vi "LINX - Servo 1 Channel my.vi"() -> ()   [LabVIEW 2017]
doc: "This example demonstrates how to control a servo using LINX."
uses:
  <vilib>/MakerHub/LINX/Public/Utilities/Open Serial.vi
  <vilib>/MakerHub/LINX/Public/Sensors/Motion/Servo/Servo Open One Channel.vi
  <vilib>/MakerHub/LINX/Public/Sensors/Motion/Servo/Servo Set Pulse Width One Channel.vi
  <vilib>/MakerHub/LINX/Public/Sensors/Motion/Servo/Servo Close One Channel.vi
  <vilib>/express/express arith-compare/Formula/XNode/ExpressFormulaBlockNode.xnode
  <vilib>/MakerHub/LINX/LMH-LINX.lvlib
  <vilib>/MakerHub/LINX/Public/Sensors/Motion/Servo/Servo.lvlib
panel:
  out "Boolean 5":bool
  out "Boolean 4":bool
  out "Boolean 3":bool
  out "Boolean 2":bool
  out "Boolean":bool
  in  "Numeric Control 4":dbl
  in  "Numeric Control 3":dbl
  in  "Soak method":string(combo)
  out "Thermometer 2":dbl(slide) scale=0.0..100.0
  out "Thermometer":dbl(slide) scale=0.0..100.0
  out "mov_ult":dbl
  out "mov1":dbl
  out "mov_for":dbl
  in  "Setpoint":dbl
  in  "Setpoint":dbl
  out "Numeric Control 2":i32
  in  "Numeric Control":i32
  out "Position":dbl(knob) scale=500.0..2500.0
  in  "Right delay":dbl
  in  "Left delay":dbl
  in  "Maximum angle":dbl(knob) scale=500.0..2500.0
  in  "Minimum angle":dbl(knob) scale=500.0..2500.0
  in  "Right velocity":dbl
  in  "Left velocity":dbl
  in  "Servo Channel":u8=2
  in  "Stop Button":bool
  in  "Serial Port":refnum<visa-resource-name>
  # "Servo Position \n(Pulse Width uS)"
  # "Servo Velocity \n(Pulse Width uS)"
  # "Hot Box"
  # "LINX Device Settings"
  # "Current temperature 1"
  # "Cycles"
  # "Servo Delay"
  # "Cold Box"
  # "Current temperature 2"
  # "Servo Live"
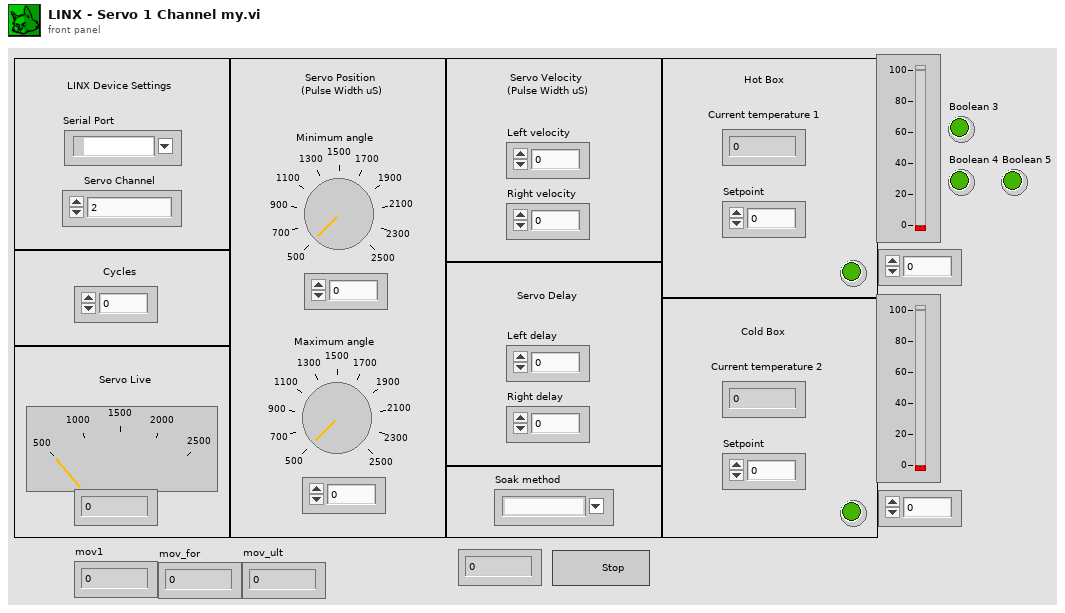
[diagram p1: front panel]
types:
  T1 = typedef "LMH-LINX.lvlib/LINX Ref.ctl" = cluster{"IO":T2, "Interface":T3, "LINX Device Config":T4}
  T2 = typedef "LMH-LINX.lvlib/Platform.ctl" = enum16{"Remote", "Local"}
  T3 = typedef "LMH-LINX.lvlib/Interface.ctl" = enum16{"Serial", "TCP"}
  T4 = typedef "LMH-LINX.lvlib/Device.lvlib/LINX Device Config.ctl" = cluster{"Interface":T3, "COM Port":refnum<visa-resource-name>, "TCP Configuration":T5, "Device Family":u8, "Device ID":u8, "Device Name":string, "TCP Ref":refnum<k5>, "Channels":T6}
  T5 = typedef "LMH-LINX.lvlib/Device.lvlib/TCP Config.ctl" = cluster{"IP Address":string, "Port":u16}
  T6 = typedef "LMH-LINX.lvlib/Channels.ctl" = cluster{"DI":u8[], "DO":u8[], "AI":u8[], "AO":u8[], "PWM":u8[], "QE":u8[], "UART":u8[], "I2C 2":u8[], "SPI":u8[], "CAN":u8[], "Servo":u8[], "AI Ref (V)":dbl, "AI Resolution (Bits)":u8, "AO Ref (V)":dbl, "AO Resolution (Bits)":u8}
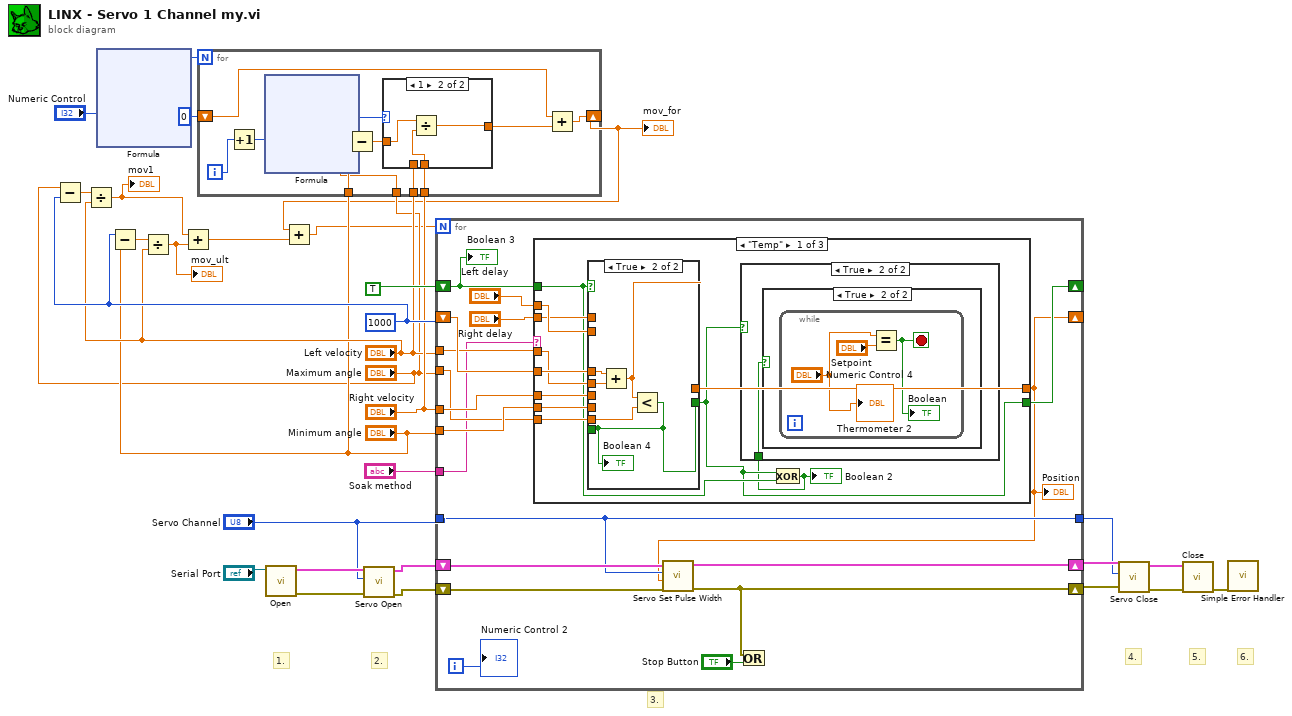
[diagram p0: block diagram]
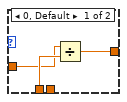
[diagram p2: hidden frame]
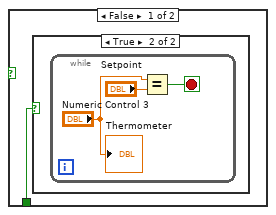
[diagram p3: hidden frame]
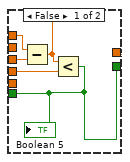
[diagram p6: hidden frame]
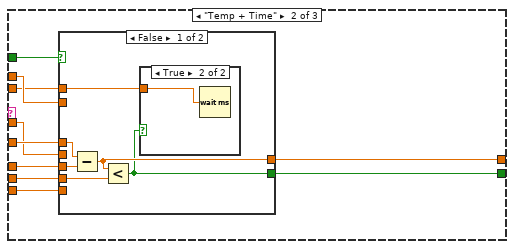
[diagram p7: hidden frame]
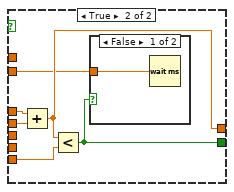
[diagram p9: hidden frame]
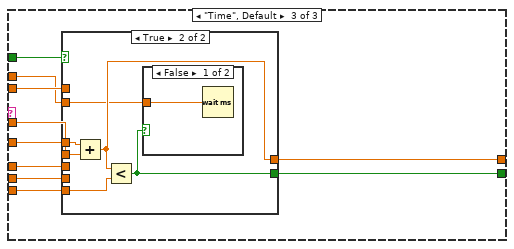
[diagram p11: hidden frame]
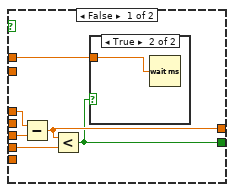
[diagram p12: hidden frame]
diagram:
  w15 = 1000
  # "6."
  # "5."
  # "4."
  # "3."
  # "2."
  # "1."
  n1 = Subtract(x="Maximum angle", y=w15) -> (x-y=w16:dbl)
  n2 = Divide(x=w16, y="Left velocity") -> (x/y=w6:dbl)
  "mov1" <- w6
  n3 = xnode "Formula"("X1"="Numeric Control") -> ("Result"=w4:i32)  [unwired: 1 in, 1 out]
  n4 = Subtract(x=w15, y="Minimum angle") -> (x-y=w14:dbl)
  n5 = Divide(x=w14, y="Left velocity") -> (x/y=w7:dbl)
  "mov_ult" <- w7
  n6 = Add(x=w6, y=w7) -> (x+y=w8:dbl)
  n7 = for {
    N: w4 -> [_]
    tunnel: "Right velocity" -> [w38]
    tunnel: "Left velocity" -> [w37]
    tunnel: "Minimum angle" -> [w31]
    tunnel: "Maximum angle" -> [w30]
    shift-right: [w32] -> w3
    shift-left: 0 -> [w34]
    i -> [w33]
    n8 = Increment(x=w33) -> (x+1=w40:i32)
    n9 = xnode "Formula"("X1"=w40) -> ("Result"=w39:i32)  [unwired: 1 in, 1 out]
    n10 = Subtract(x=w30, y=w31) -> (x-y=w36:dbl)
    n11 = case shown="1" w39 {
      tunnel: w38 -> [_ w44]
      tunnel: w37 -> [w43 _]
      tunnel: w36 -> [w42 w46]
      tunnel: [w41 w45] -> w35
      frame 0, Default {
        n12 = Divide(x=w42, y=w43) -> (x/y=w41:dbl)
      }
      frame 1 {
        n13 = Divide(x=w46, y=w44) -> (x/y=w45:dbl)
      }
    }
    n14 = Add(x=w34, y=w35) -> (x+y=w32:dbl)
  }
  "mov_for" <- w3
  n15 = call-poly <vilib>:"Open.vi"("Serial Port"="Serial Port") -> ("Error Out"=w28:errorcluster, "LINX Resource"=w27:T1)  [unwired: 8 in, 1 out]
  n16 = Add(x=w3, y=w8) -> (x+y=w2:dbl)
  n17 = call-poly <vilib>:"Servo Open.vi"("Error In"=w28, "Servo Channel"="Servo Channel", "LINX Resource"=w27) -> ("Error Out"=w26:errorcluster, "LINX Resource"=w25:T1)  [unwired: 7 in]
  n18 = for {
    N: w2 -> [_]
    shift-right: [w70] -> w19
    shift-left: w26 -> [w71]
    tunnel: "Servo Channel" -> [w67]
    shift-right: [w68] -> w22
    shift-left: w25 -> [w69]
    tunnel: [w67] -> w18
    shift-right: [w65] -> _
    shift-left: TRUE -> [w55]
    shift-right: [w59] -> _
    shift-left: w15 -> [w66]
    tunnel: "Minimum angle" -> [w63]
    tunnel: "Right velocity" -> [w62]
    tunnel: "Maximum angle" -> [w61]
    tunnel: "Left velocity" -> [w60]
    tunnel: "Soak method" -> [w58]
    i -> [w64]
    n19 = case shown="\"Temp\"" w58 {
      tunnel: w66 -> [w80 w106 w135]
      tunnel: [w74 w110 w134] -> w65
      tunnel: w55 -> [w75 w109 w133]
      tunnel: w63 -> [w77 w103 w132]
      tunnel: w62 -> [w78 w104 w131]
      tunnel: w61 -> [w76 w102 w130]
      tunnel: w60 -> [w79 w105 w129]
      tunnel: [w83 w111 w128] -> w59
      tunnel: "Right delay" -> [w81 w107 w127]
      tunnel: "Left delay" -> [w82 w108 w126]
      frame "Temp" {
        n20 = case shown="True" w75 {
          tunnel: w80 -> [w96 w101]
          tunnel: [w93 w98] -> w83
          tunnel: [w92 w97] -> w74
          tunnel: w79 -> [_ w100]
          tunnel: w76 -> [_ w99]
          tunnel: w78 -> [w95 _]
          tunnel: w77 -> [w94 _]
          tunnel: w82 -> [_ _]
          tunnel: w81 -> [_ _]
          tunnel: [w92 w97] -> _
          frame False {
            n21 = Subtract(x=w96, y=w95) -> (x-y=w93:dbl)
            n22 = Less?(x=w93, y=w94) -> (x < y?=w92:bool)
            "Boolean 5" <- w92
          }
          frame True {
            n23 = Add(x=w101, y=w100) -> (x+y=w98:dbl)
            n24 = Less?(x=w98, y=w99) -> (x < y?=w97:bool)
            "Boolean 4" <- w97
          }
        }
        n25 = Exclusive Or(1:w75, 2:w74) -> (0:w73:bool)
        "Boolean 2" <- w73
        n26 = case shown="True" w74 {
          tunnel: w73 -> [w84 w88]
          frame False {
            n27 = case shown="True" w84 {
              frame False {
              }
              frame True {
                n28 = while {
                  stop <- w85 stop-if-true
                  n29 = Equal?(x="Numeric Control 3", y="Setpoint") -> (x = y?=w85:bool)
                  "Thermometer" <- "Numeric Control 3"
                }
              }
            }
          }
          frame True {
            n30 = case shown="True" w88 {
              frame False {
              }
              frame True {
                n31 = while {
                  stop <- w89 stop-if-true
                  n32 = Equal?(x="Numeric Control 4", y="Setpoint") -> (x = y?=w89:bool)
                  "Boolean" <- w89
                  "Thermometer 2" <- "Numeric Control 4"
                }
              }
            }
          }
        }
      }
      frame "Temp + Time" {
        n33 = case shown="False" w109 {
          tunnel: w106 -> [w117 w124]
          tunnel: [w114 w121] -> w111
          tunnel: [w113 w120] -> w110
          tunnel: w105 -> [_ w123]
          tunnel: w102 -> [_ w122]
          tunnel: w104 -> [w116 _]
          tunnel: w103 -> [w115 _]
          tunnel: w108 -> [_ w119]
          tunnel: w107 -> [w112 _]
          frame False {
            n34 = Subtract(x=w117, y=w116) -> (x-y=w114:dbl)
            n35 = Less?(x=w114, y=w115) -> (x < y?=w113:bool)
            n36 = case shown="True" w113 {
              tunnel: w112 -> [_ w118]
              frame False {
              }
              frame True {
                n37 = Wait (ms)(milliseconds to wait=w118) -> ()  [unwired: 1 out]
              }
            }
          }
          frame True {
            n38 = Add(x=w124, y=w123) -> (x+y=w121:dbl)
            n39 = Less?(x=w121, y=w122) -> (x < y?=w120:bool)
            n40 = case shown="False" w120 {
              tunnel: w119 -> [w125 _]
              frame False {
                n41 = Wait (ms)(milliseconds to wait=w125) -> ()  [unwired: 1 out]
              }
              frame True {
              }
            }
          }
        }
      }
      frame "Time", Default {
        n42 = case shown="True" w133 {
          tunnel: w135 -> [w141 w148]
          tunnel: [w138 w145] -> w128
          tunnel: [w137 w144] -> w134
          tunnel: w129 -> [_ w147]
          tunnel: w130 -> [_ w146]
          tunnel: w131 -> [w140 _]
          tunnel: w132 -> [w139 _]
          tunnel: w126 -> [_ w143]
          tunnel: w127 -> [w136 _]
          frame False {
            n43 = Subtract(x=w141, y=w140) -> (x-y=w138:dbl)
            n44 = Less?(x=w138, y=w139) -> (x < y?=w137:bool)
            n45 = case shown="True" w137 {
              tunnel: w136 -> [_ w142]
              frame False {
              }
              frame True {
                n46 = Wait (ms)(milliseconds to wait=w142) -> ()  [unwired: 1 out]
              }
            }
          }
          frame True {
            n47 = Add(x=w148, y=w147) -> (x+y=w145:dbl)
            n48 = Less?(x=w145, y=w146) -> (x < y?=w144:bool)
            n49 = case shown="False" w144 {
              tunnel: w143 -> [w149 _]
              frame False {
                n50 = Wait (ms)(milliseconds to wait=w149) -> ()  [unwired: 1 out]
              }
              frame True {
              }
            }
          }
        }
      }
    }
    "Position" <- w59
    n51 = call-poly <vilib>:"Servo Set Pulse Width.vi"("Error In"=w71, "Pulse Width (uS)"=w59, "Servo Channel"=w67, "LINX Resource"=w69) -> ("Error Out"=w70:errorcluster, "LINX Resource"=w68:T1)  [unwired: 6 in]
    n52 = Or(x=w70, y="Stop Button") -> ()  [unwired: 1 out]
    "Numeric Control 2" <- w64
    "Boolean 3" <- w55
  }
  n53 = call-poly <vilib>:"Servo Close.vi"("Error In"=w19, "Servo Channel"=w18, "LINX Resource"=w22) -> ("Error Out"=w20:errorcluster, "LINX Resource"=w21:T1)  [unwired: 7 in]
  n54 = call <vilib>:"Close.vi"("Error In"=w20, "LINX Resource"=w21) -> ("Error Out"=w23:errorcluster)  [unwired: 9 in]
  n55 = call <vilib>:"Simple Error Handler.vi"("error in (no error)"=w23) -> ()  [unwired: 4 in, 5 out]
